vi "fpga_LP2 Filter_engineunit0 (M Class_50Hz).vi"(0 "input data":fxp<+/-,32,5>, 1 "ACC_Load":bool, 7 "coefficients":fxp<+/-,19,-3>[](array[numeric])=[0.0], 11 "opState":T1) -> (4 "output data":fxp<+/-,32,6>)   [LabVIEW 2013, in "NI_EP_PMU_FPGA.lvlib"]
uses:
  <vilib>/addons/Electrical Power/PMU/NI_EP_PMU_FPGA.lvlib
  <vilib>/rvi/FXPMathLib/basic elements/FxpIntAccumulator/subVIs/nifxpmath_IntAccumulator_SimConfig.ctl
  <vilib>/rvi/FXPMathLib/basic elements/FxpIntAccumulator/simVIs/DllFxpIntAccumulator_sub.vi
  <vilib>/rvi/FXPMathLib/basic elements/FxpIntAccumulator/XNode/nifxpmath_IntAccumulator.xnode
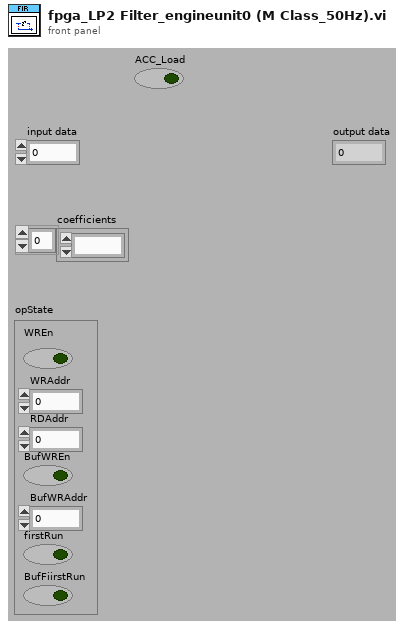
[diagram p1: front panel]
types:
  T1 = cluster{"WREn":bool, "WRAddr":fxp<+,14,14>, "RDAddr":fxp<+,14,14>, "BufWREn":bool, "BufWRAddr":fxp<+,14,14>, "firstRun":bool, "BufFiirstRun":bool}
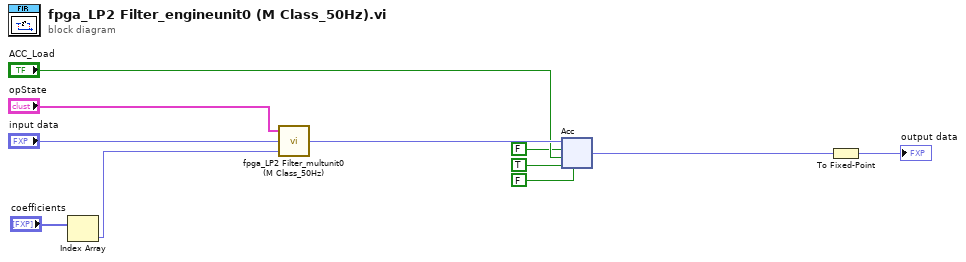
[diagram p0: block diagram]
diagram:
  n1 = Index Array ("CoefExpander")(array="coefficients") -> (element=w4:fxp<+/-,19,-3>)  [unwired: 1 in]
  n2 = call <vilib>:"fpga_LP2 Filter_multunit0 (M Class_50Hz).vi"("opState"="opState", "x"="input data", "coef"=w4) -> ("y"=w11:fxp<+/-,48,6>)  [unwired: 5 in, 1 out]
  n3 = xnode ("Acc")("x"=w11, "load (F)"="ACC_Load", "is sub? (F)"=FALSE ("is sub?"), "enable (T)"=TRUE ("enable"), "carry-in/inverted borrow-in (F)"=FALSE ("carry-in/no borrow-in")) -> ("s"=w9:fxp<+/-,48,6>)  [unwired: 1 out]
  n4 = To Fixed-Point ("toOutput")(number=w9) -> (fixed-point=→"output data":fxp<+/-,32,6>)  [unwired: 1 out]
